vi "Last Updated Comparison.vi"(8 "SR Cluster 2 in":T1 {"Creation Date" format="%<%x>T"; "Last Updated" format="%<%x>T"}, 9 "SR Cluster 1 in":T1 {"Creation Date" format="%<%x>T"; "Last Updated" format="%<%x>T"}, 10 "flip? in":bool, 11 "equal? in":bool) -> (0 "SR Cluster 2 out":T1 {"Creation Date" format="%<%x>T"; "Last Updated" format="%<%x>T"}, 1 "SR Cluster 1 out":T1 {"Creation Date" format="%<%x>T"; "Last Updated" format="%<%x>T"}, 2 "flip? out":bool, 3 "equal? out":bool)   [LabVIEW 2018]
uses:
  Type Defs/SR Cluster.ctl
  Type Defs/SR Status.ctl
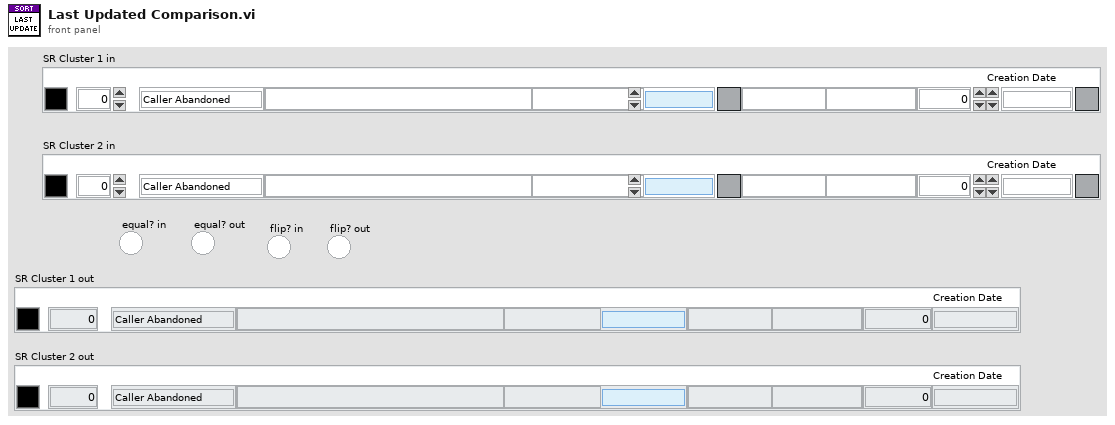
[diagram p1: front panel]
types:
  T1 = typedef "SR Cluster.ctl" = cluster{"Color":u32, "SR Number":i32, "SR Status":T2, "Name":string, "Summary":string, "Last Updated":timestamp, "SR Type":string, "Service Level":string, "Days Open":dbl, "Creation Date":timestamp}
  T2 = typedef "SR Status.ctl" = enum16{"Caller Abandoned", "Created in Error", "Expired", "Forum Resolved AE", "Forum Resolved Customer", "IN WORK", "IN WORK Collab with AES", "IN WORK Collab with PSE", "IN WORK Collab with SE", "IN WORK Customer Added Note", "IN WORK Escalation", "IN WORK Wait on Customer", "Open", "Potentially Resolved", "Presumed Resolved", "RMA Approved for Return", "Resolved", "Passed Off"}
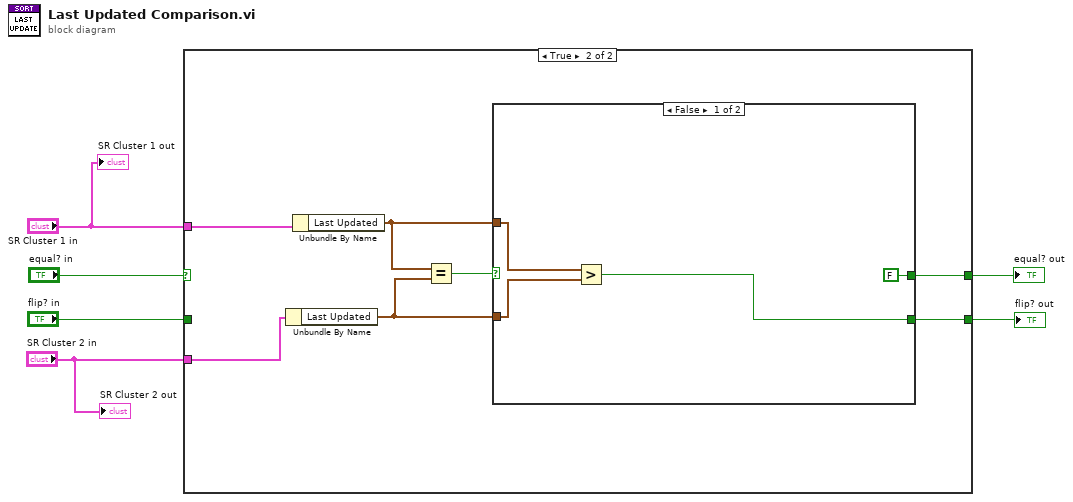
[diagram p0: block diagram]
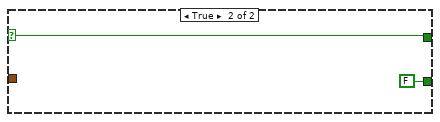
[diagram p3: hidden frame]
diagram:
  n1 = case shown="True" "equal? in" {
    selector: "equal? in" -> [w7 _]
    tunnel: [w8 w15] -> w6
    tunnel: "flip? in" -> [w8 _]
    tunnel: [w7 w13] -> w3
    tunnel: "SR Cluster 2 in" -> [_ w10]
    tunnel: "SR Cluster 1 in" -> [_ w9]
    frame False {
    }
    frame True {
      n2 = Unbundle By Name(w10) -> ("Last Updated"=w12:timestamp)
      n3 = Unbundle By Name(w9) -> ("Last Updated"=w11:timestamp)
      n4 = Equal?(x=w11, y=w12) -> (x = y?=w14:bool)
      n5 = case shown="False" w14 {
        selector: w14 -> [_ w20]
        tunnel: [w19 FALSE] -> w15
        tunnel: [FALSE w20] -> w13
        tunnel: w12 -> [w17 _]
        tunnel: w11 -> [w18 _]
        frame False {
          n6 = Greater?(x=w18, y=w17) -> (0:w19:bool)
        }
        frame True {
        }
      }
    }
  }
  "equal? out" <- w3
  "flip? out" <- w6
  "SR Cluster 2 out" <- "SR Cluster 2 in"
  "SR Cluster 1 out" <- "SR Cluster 1 in"
